vi "Get Network Endpoint Enqueuer.vi"(8 "error in":errorcluster, 11 "Study Actor in":refnum<class "Study Actor.lvclass">) -> (0 "error out":errorcluster, 1 "Connected":bool, 2 "Network Endpoint Enqueuer":refnum<class "Message Enqueuer.lvclass">, 3 "Study Actor out":refnum<class "Study Actor.lvclass">)   [LabVIEW 2024, in "Study Actor.lvlib" / "Study Actor.lvclass"]
uses:
  Study Actor.lvclass
  Study Actor.lvclass/Study Actor.ctl
  Nested Actors Study.ctl
  <vilib>/ActorFramework/Message Enqueuer/Message Enqueuer.lvclass
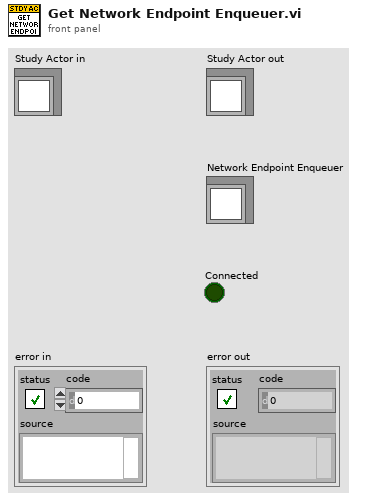
[diagram p1: front panel]
types:
  T1 = typedef "Nested Actors Study.ctl" = enum16{"Series", "Network Endpoint"}
  T2 = map{u16, refnum<class "Message Enqueuer.lvclass">}
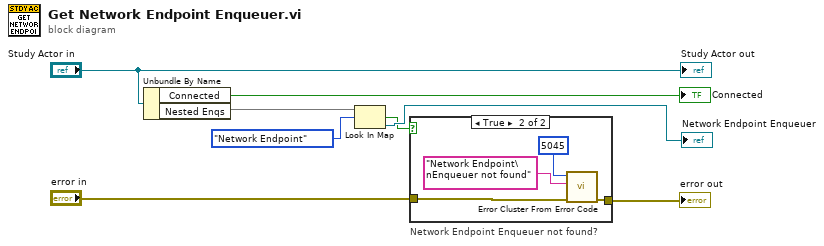
[diagram p0: block diagram]
diagram:
  n1 = Unbundle By Name("Study Actor in") -> ("Connected"=→"Connected":bool, "Nested Enqs"=w3:T2)
  n2 = Look In Map(map=w3, key=Nested_Actors_Study."Network Endpoint" ("Nested Actors Study")) -> (key not found?=w2:bool, value=→"Network Endpoint Enqueuer":refnum<class "Message Enqueuer.lvclass">)  [unwired: 1 in]
  n3 = case "Network Endpoint Enqueuer not found?" shown="True" w2 {
    tunnel: "error in" -> [w9 w13]
    tunnel: [w9 w12] -> w7
    frame False {
    }
    frame True {
      n4 = call <vilib>:"Error Cluster From Error Code.vi"("error in (no error)"=w13, "error message (\"\")"="Network Endpoint\nEnqueuer not found" ("error message (\"\")"), "error code (0)"=5045) -> ("error out"=w12:errorcluster)  [unwired: 6 in]
    }
  }
  "error out" <- w7
  "Study Actor out" <- "Study Actor in"
